vi "ST Rotate Joint.vi"(5 "error in (no error)":errorcluster, 6 "Radians":dbl, 7 "Joint to rotate":string(combo)="WAIST", 8 "VISA resource name":refnum<visa-resource-name>) -> (0 "error out":errorcluster, 1 "String Received":string, 2 "Ready and OK":bool, 3 "VISA resource name out":refnum<visa-resource-name>, 4 "Result Code":i32)   [LabVIEW 2009]
doc: "This VI will rotate a single joint, using joint mode. \n\nSelect the joint to be rotated and the angle in radians, - indicates reverse."
panel:
  # "THIS VI ROTATES THE CHOSEN JOINT THE NUMBER OF RADIANS PASSED"
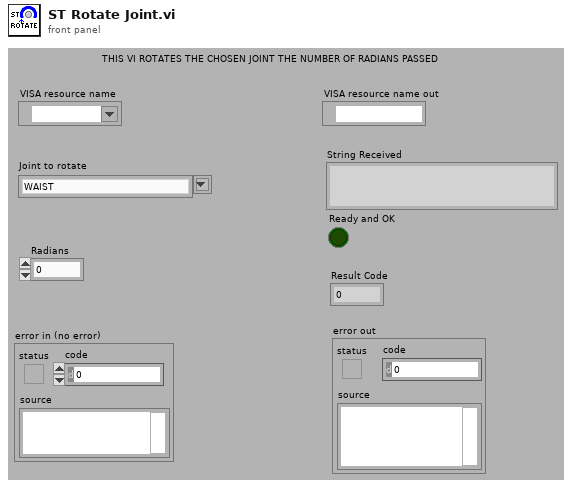
[diagram p1: front panel]
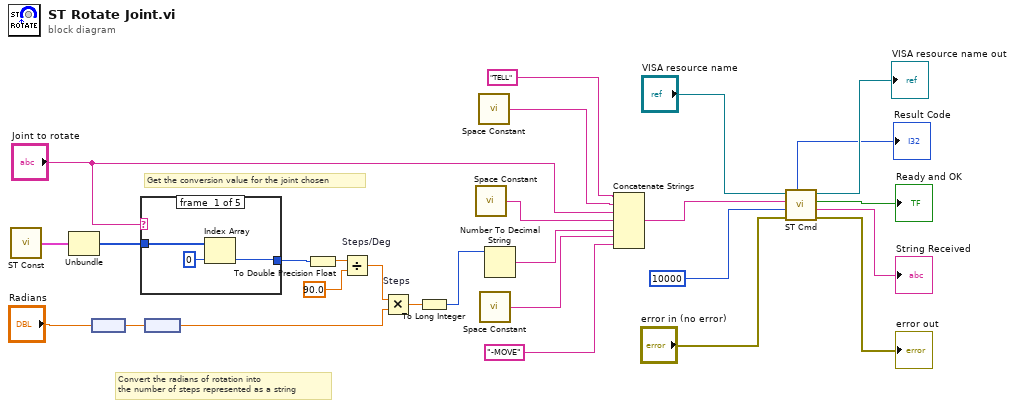
[diagram p0: block diagram]
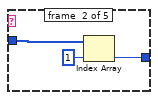
[diagram p2: hidden frame]
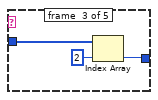
[diagram p3: hidden frame]
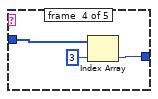
[diagram p4: hidden frame]
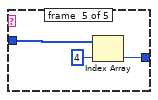
[diagram p5: hidden frame]
diagram:
  # "Get the conversion value for the joint chosen"
  # "Convert the radians of rotation into \nthe number of steps represented as a string"
  n1 = call "ST Const.vi"() -> ("Robot Constants"=w13:cluster{i32[], i32[], dbl[]})
  n2 = Unbundle(w13) -> (w11:i32[])  [unwired: 2 out]
  n3 = node("Radians") -> (w8:dbl[unit])
  n4 = case shown="\"WAIST\", Default" "Joint to rotate" {
    tunnel: w11 -> [w30 w32 w35 w38 w41]
    tunnel: [w28 w31 w34 w37 w40] -> w3
    frame #0 {
      n5 = Index Array(array=w30, index=0) -> (element=w28:i32)
    }
    frame #1 {
      n6 = Index Array(array=w32, index=1) -> (element=w31:i32)
    }
    frame #2 {
      n7 = Index Array(array=w35, index=2) -> (element=w34:i32)
    }
    frame #3 {
      n8 = Index Array(array=w38, index=3) -> (element=w37:i32)
    }
    frame #4 {
      n9 = Index Array(array=w41, index=4) -> (element=w40:i32)
    }
  }
  n10 = node(w8) -> (w6:dbl)
  n11 = To Double Precision Float(number=w3) -> (double precision float=w9:dbl)
  n12 = Divide "Steps/Deg"(x=w9, y=90.0) -> (x/y=w7:dbl)
  n13 = Multiply "Steps"(x=w7, y=w6) -> (x*y=w5:dbl)
  n14 = To Long Integer(number=w5) -> (32bit integer=w2:i32)
  n15 = call <vilib>:"Space Constant.vi"() -> ("String"=w16:string)
  n16 = call <vilib>:"Space Constant.vi"() -> ("String"=w17:string)
  n17 = call <vilib>:"Space Constant.vi"() -> ("String"=w14:string)
  n18 = Number To Decimal String(number=w2) -> (decimal integer string=w1:string)  [unwired: 1 in]
  n19 = Concatenate Strings("TELL", w17, "Joint to rotate", w16, w1, w14, "-MOVE") -> (w18:string)
  n20 = call "ST Cmd.vi"("error in (no error)"="error in (no error)", "Time Out"=10000, "Command String"=w18, "VISA resource name"="VISA resource name") -> ("error out"=→"error out":errorcluster, "String Received"=→"String Received":string, "Ready and OK"=→"Ready and OK":bool, "VISA resource name out"=→"VISA resource name out":refnum<visa-resource-name>, "Result Code"=→"Result Code":i32)
